vi "IR Cube Pull.vi"(7 "Cube?":bool, 8 "Constant Pull Rate":dbl, 9 "Right Arm":dbl, 10 "Left Arm":dbl, 11 "Manual Roller Power":dbl) -> (1 "Right Arm Out":dbl, 3 "Left Arm Out":dbl)   [LabVIEW 2017]
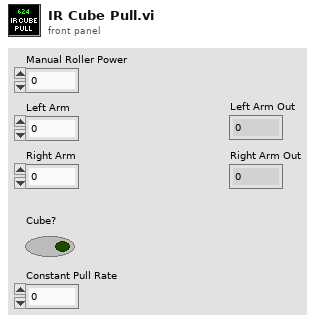
[diagram p1: front panel]
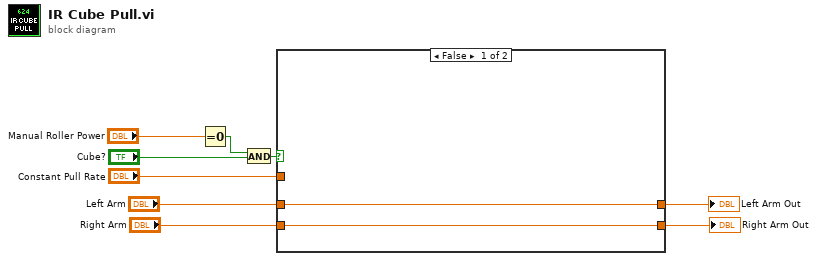
[diagram p0: block diagram]
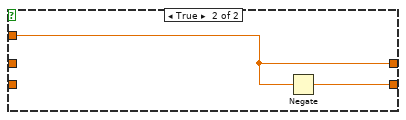
[diagram p2: hidden frame]
diagram:
  n1 = Equal To 0?(x="Manual Roller Power") -> (x = 0?=w8:bool)
  n2 = And(x=w8, y="Cube?") -> (x .and. y?=w9:bool)
  n3 = case shown="False" w9 {
    tunnel: "Constant Pull Rate" -> [_ w12]
    tunnel: [w11 w12] -> w4
    tunnel: [w10 w13] -> w3
    tunnel: "Left Arm" -> [w11 _]
    tunnel: "Right Arm" -> [w10 _]
    frame False {
    }
    frame True {
      n4 = Negate(x=w12) -> (-x=w13:dbl)
    }
  }
  "Left Arm Out" <- w4
  "Right Arm Out" <- w3
